vi "例10.6  利用高层函数连续采集图像（grab）.vi"() -> ()   [LabVIEW 2017]
doc: "The Grab VI acquires images continuously and displays the images in an image control using high-level acquisition VIs. A grab is appropriate for high-speed applications in which you need to process only one image at a time."
uses:
  <vilib>/userdefined/High Color/IMAQdx.ctl
  <vilib>/vision/driver/NI_Vision_Acquisition_Software.lvlib
panel:
  in  "Camera Name":T1
  out "Buffer Number":u32
  out "Image":T2(plugin-control)
  in  "stop":bool
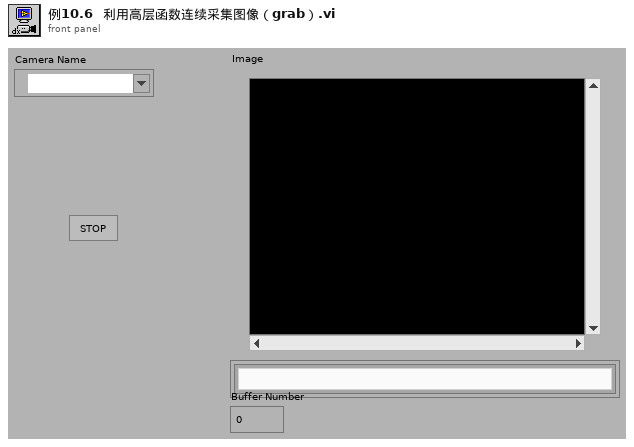
[diagram p1: front panel]
types:
  T1 = typedef "IMAQdx.ctl" = refnum<k21>
  T2 = typedef "IMAQ Image.ctl" = refnum<image>
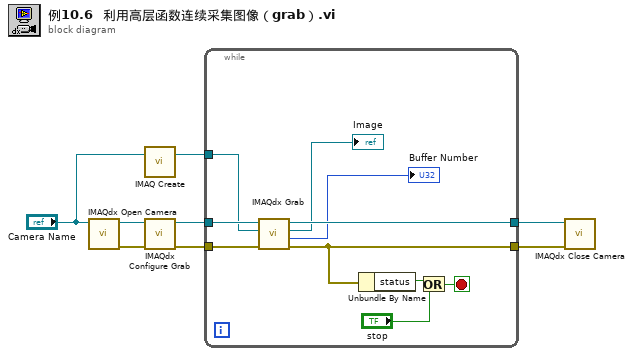
[diagram p0: block diagram]
diagram:
  n1 = call <vilib>:"IMAQdx Open Camera.vi"("Session In"="Camera Name") -> ("error out"=w3:errorcluster, "Session Out"=w2:T1)  [unwired: 2 in, 7 out]
  n2 = call "IMAQ Create"("Image Name"="Camera Name") -> ("New Image"=w8:T2)  [unwired: 3 in, 2 out]
  n3 = call <vilib>:"IMAQdx Configure Grab.vi"("error in"=w3, "Session In"=w2) -> ("error out"=w6:errorcluster, "Session Out"=w7:T1)  [unwired: 8 out]
  n4 = while {
    tunnel: [w12] -> w5
    tunnel: w6 -> [w14]
    tunnel: w7 -> [w15]
    tunnel: [w11] -> w4
    tunnel: w8 -> [w13]
    stop <- w18 stop-if-true
    n5 = call <vilib>:"IMAQdx Grab.vi"("error in"=w14, "Image In"=w13, "Session In"=w15) -> ("error out"=w11:errorcluster, "Buffer Number Out"=→"Buffer Number":u32, "Image Out"=→"Image":T2, "Session Out"=w12:T1)  [unwired: 1 in, 4 out]
    n6 = Unbundle By Name(w11) -> ("status"=w17:bool)
    n7 = Or(x=w17, y="stop") -> (x .or. y?=w18:bool)
  }
  n8 = call <vilib>:"IMAQdx Close Camera.vi"("error in"=w4, "Session In"=w5) -> ()  [unwired: 10 out]
